vi "LVProjectShortcut_OnShortcutView.vi"(8 "error in":errorcluster, 11 "Object":T1) -> (0 "error out":errorcluster)   [LabVIEW 2017, in "LVProject Shortcut.lvlib"]
uses:
  <resource>/Framework/Providers/API/ItemRef.ctl
  LVProject Shortcut.lvlib
  <vilib>/Utility/lvfile.llb/NI_FileType.lvlib
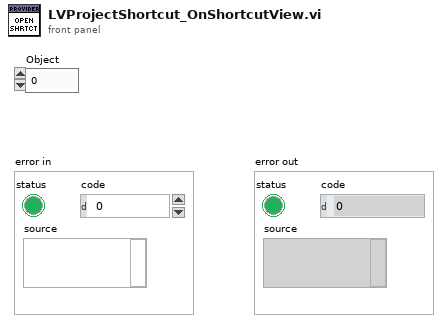
[diagram p1: front panel]
types:
  T1 = typedef "ItemRef.ctl" = u64
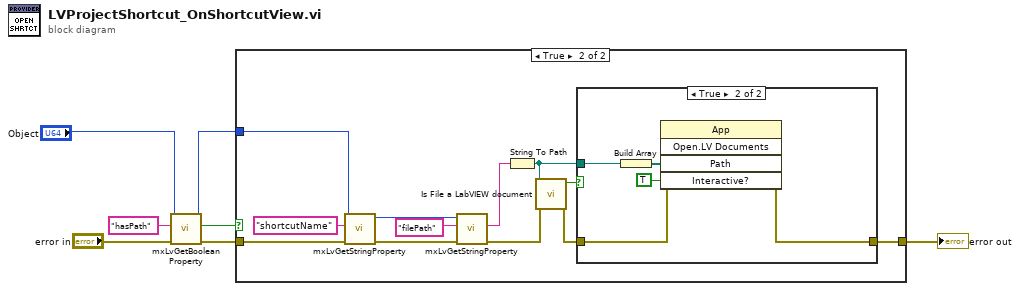
[diagram p0: block diagram]
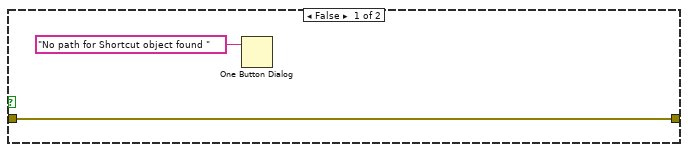
[diagram p2: hidden frame]
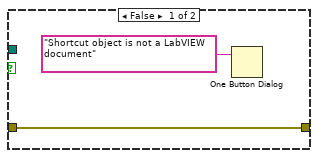
[diagram p3: hidden frame]
diagram:
  n1 = call <resource>:"mxLvGetBooleanProperty.vi"("error in"="error in", "Tag"="hasPath", "Item"="Object") -> ("error out"=w3:errorcluster, "Value"=w2:bool, "Item"=w4:T1)  [unwired: 6 in]
  n2 = case shown="True" w2 {
    tunnel: w4 -> [_ w15]
    tunnel: w3 -> [w9 w21]
    tunnel: [w9 w14] -> w1
    frame False {
      n3 = One Button Dialog(message="No path for Shortcut object found ") -> ()  [unwired: 1 in, 1 out]
    }
    frame True {
      n4 = call <resource>:"mxLvGetStringProperty.vi"("Error In"=w21, "Tag"="shortcutName", "Item"=w15) -> ("Error Out"=w20:errorcluster, "Item"=w17:T1)  [unwired: 6 in, 1 out]
      n5 = call <resource>:"mxLvGetStringProperty.vi"("Error In"=w20, "Tag"="filePath", "Item"=w17) -> ("Error Out"=w10:errorcluster, "Value"=w16:string)  [unwired: 6 in, 1 out]
      n6 = String To Path(string=w16) -> (path=w13:path)
      n7 = call <vilib>:"Is File a LabVIEW document.vi"("error in (no error)"=w10, "path"=w13) -> ("error out"=w11:errorcluster, "Is LabVIEW document?"=w12:bool)  [unwired: 8 in]
      n8 = case shown="True" w12 {
        tunnel: w11 -> [w23 w27]
        tunnel: [w23 w26] -> w14
        tunnel: w13 -> [_ w24]
        frame False {
          n9 = One Button Dialog(message="Shortcut object is not a LabVIEW document") -> ()  [unwired: 1 in, 1 out]
        }
        frame True {
          n10 = Build Array(w24) -> (w28:path[])
          n11 = invoke class="App" method="Open.LV Documents"(error in=w27, "Path"=w28, "Interactive?"=TRUE) -> (error out=w26:errorcluster)  [unwired: 2 in, 4 out]
        }
      }
    }
  }
  "error out" <- w1
